vi "tt20_free_correlation.vi"(8 "error in (no error)":errorcluster, 11 "tt20 in":refnum<class "tt20.lvclass">) -> (0 "error out":errorcluster, 3 "tt20 out":refnum<class "tt20.lvclass">)   [LabVIEW 2015, in "tt20.lvclass"]
uses:
  tt20.lvclass
  tt20.lvclass/tt20.ctl
  C:/Users/MX-Microscope/Documents/LabVIEW Data/lvoop_campus_2018/Detector_Class/Swabian/time_tagger_vis/TTCSharp32.dll
  time_tagger_vis/TTCSharp32.dll
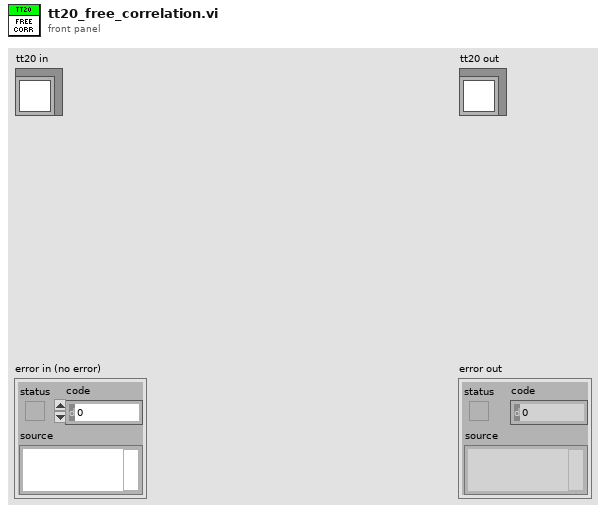
[diagram p1: front panel]
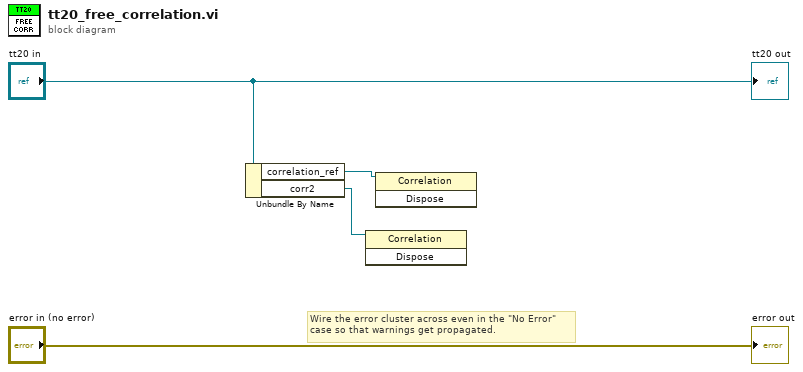
[diagram p0: block diagram]
diagram:
  # "Wire the error cluster across even in the \"No Error\"\ncase so that warnings get propagated."
  n1 = Unbundle By Name("tt20 in") -> ("correlation_ref"=w2:refnum<k24>, "corr2"=w1:refnum<k24>)
  n2 = invoke class="Correlation" method="Dispose"(reference=w1) -> ()  [unwired: 2 in, 3 out]
  n3 = invoke class="Correlation" method="Dispose"(reference=w2) -> ()  [unwired: 2 in, 3 out]
  "error out" <- "error in (no error)"
  "tt20 out" <- "tt20 in"
